vi "Filter and Sort Items.vi"(5 "Sort Info":T5={"Sort Column"=enum."Description", "Ascending?"=FALSE, "Enabled?"=FALSE}, 7 "Filter Info":T7={"Filter Column"=enum."Description", "Filter Type"=enum."Contains", "Filter Value"="", "New Data?"=FALSE, "Enabled?"=FALSE}, 10 "New VI Data":T1[](array[typedef]), 11 "Saved VI Data":T1[](array[typedef])) -> (1 "Displayed Indices":i32[](array[numeric]), 2 "New VI Data out":T1[](array[typedef]), 3 "Saved VI Data out":T1[](array[typedef]))   [LabVIEW 2023, in "VI Properties Editor.lvlib"]
doc: "Filters <B>Saved VI Data</B> according to <B>Filter</B>."
uses:
  VI Properties Editor.lvlib
  CTLs/VI Data.ctl
  CTLs/VI Properties.ctl
  <vilib>/picture/picture.llb/imagedata.ctl
  CTLs/Control Properties.ctl
  CTLs/Filter Info.ctl
  CTLs/Column Name.ctl
  CTLs/Filter Type.ctl
  CTLs/Sort Info.ctl
  <vilib>/regexp/Match Regular Expression.xnode
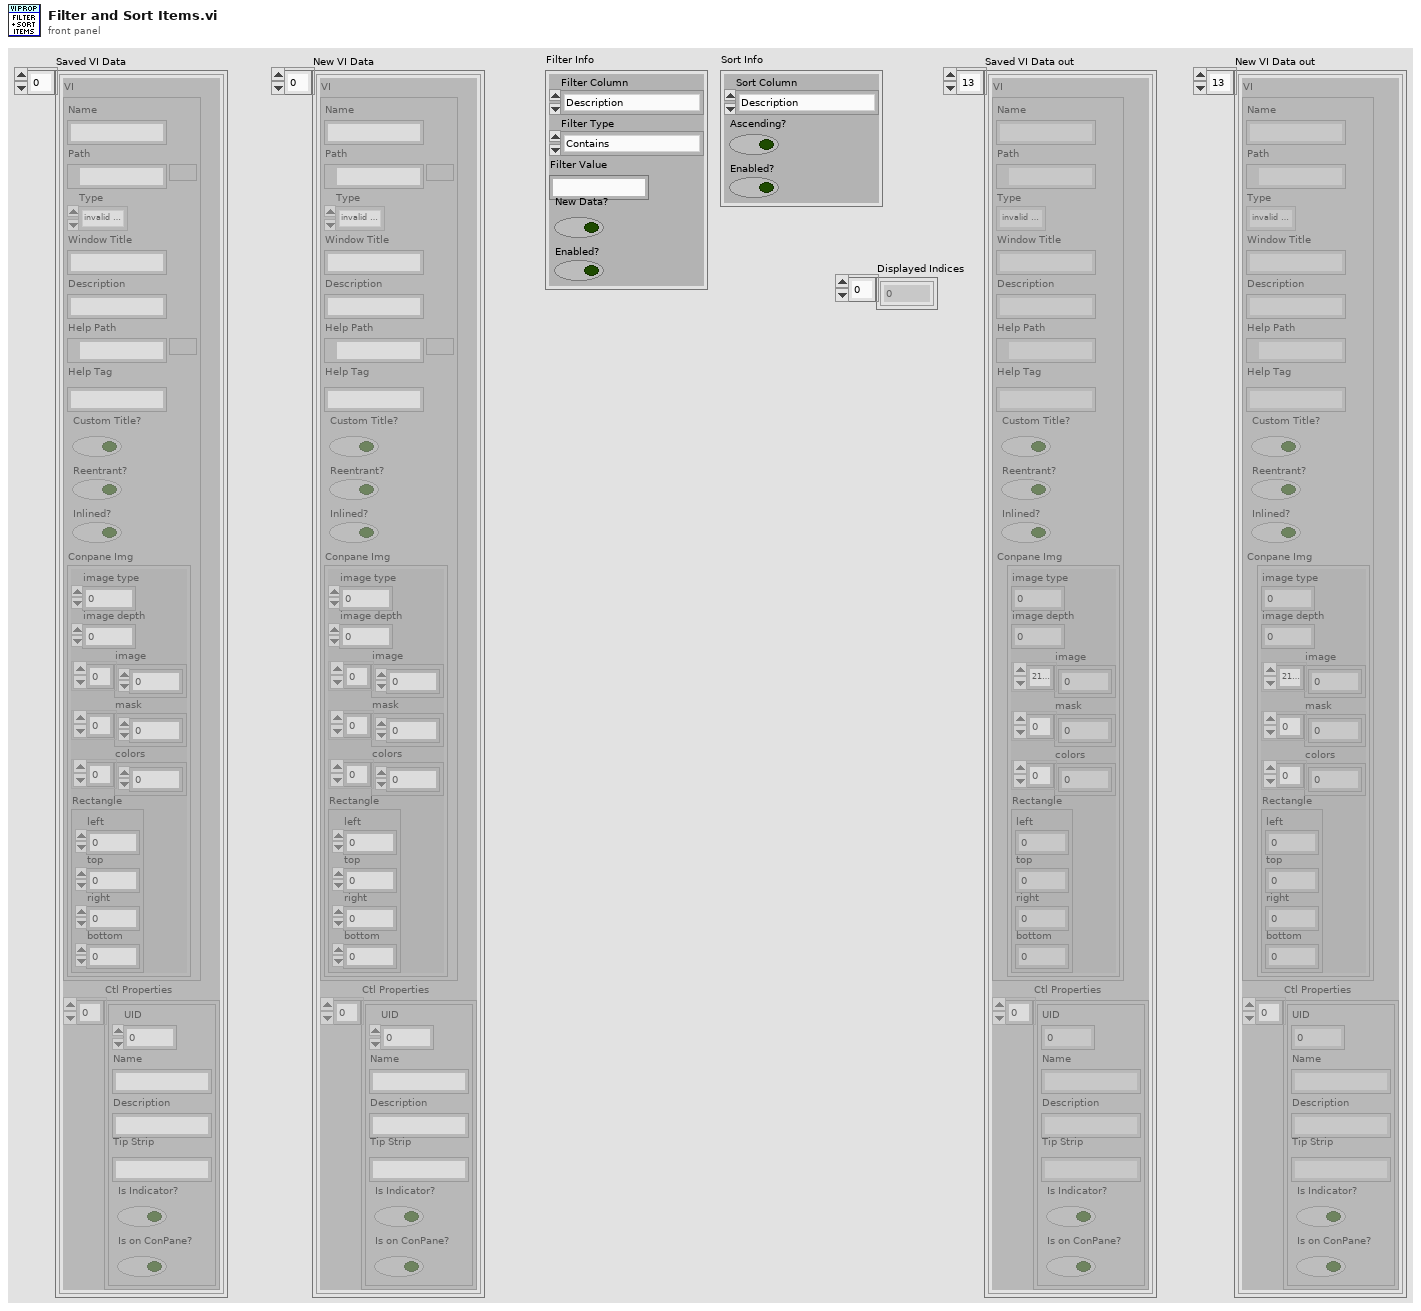
[diagram p1: front panel]
types:
  T1 = typedef "VI Properties Editor.lvlib/VI Data.ctl" = cluster{"VI":T2, "Ctl Properties":T4[]}
  T2 = typedef "VI Properties Editor.lvlib/VI Properties.ctl" = cluster{"Name":string, "Path":path, "Type":enum32{"invalid VI type", "Standard VI", "Control VI", "Global VI", "Polymorphic VI", "Configuration VI", "SubSystem", "Facade VI", "Method VI", "Statechart Diagram VI"}, "Window Title":string, "Description":string, "Help Path":path, "Help Tag":string, "Custom Title?":bool, "Reentrant?":bool, "Inlined?":bool, "Conpane Img":T3}
  T3 = typedef "imagedata.ctl" = cluster{"image type":i32, "image depth":i32, "image":u8[], "mask":u8[], "colors":u32[], "Rectangle":cluster{"left":i16, "top":i16, "right":i16, "bottom":i16}}
  T4 = typedef "VI Properties Editor.lvlib/Control Properties.ctl" = cluster{"UID":i32, "Name":string, "Description":string, "Tip Strip":string, "Is Indicator?":bool, "Is on ConPane?":bool}
  T5 = typedef "VI Properties Editor.lvlib/Sort Info.ctl" = cluster{"Sort Column":T6, "Ascending?":bool, "Enabled?":bool}
  T6 = typedef "VI Properties Editor.lvlib/Column Name.ctl" = enum16{"Name", "Path", "Type", "Window Title", "Description", "Help Path", "Help Tag", "Custom Title?", "Reentrant?", "Inlined?"}
  T7 = typedef "VI Properties Editor.lvlib/Filter Info.ctl" = cluster{"Filter Column":T6, "Filter Type":T8, "Filter Value":string, "New Data?":bool, "Enabled?":bool}
  T8 = typedef "VI Properties Editor.lvlib/Filter Type.ctl" = enum16{"Contains", "Equals", "Starts with", "Ends with", "Does not contain", "Does not equal", "Is empty", "Is not empty"}
  T9 = enum32{"invalid VI type", "Standard VI", "Control VI", "Global VI", "Polymorphic VI", "Configuration VI", "SubSystem", "Facade VI", "Method VI", "Statechart Diagram VI"}
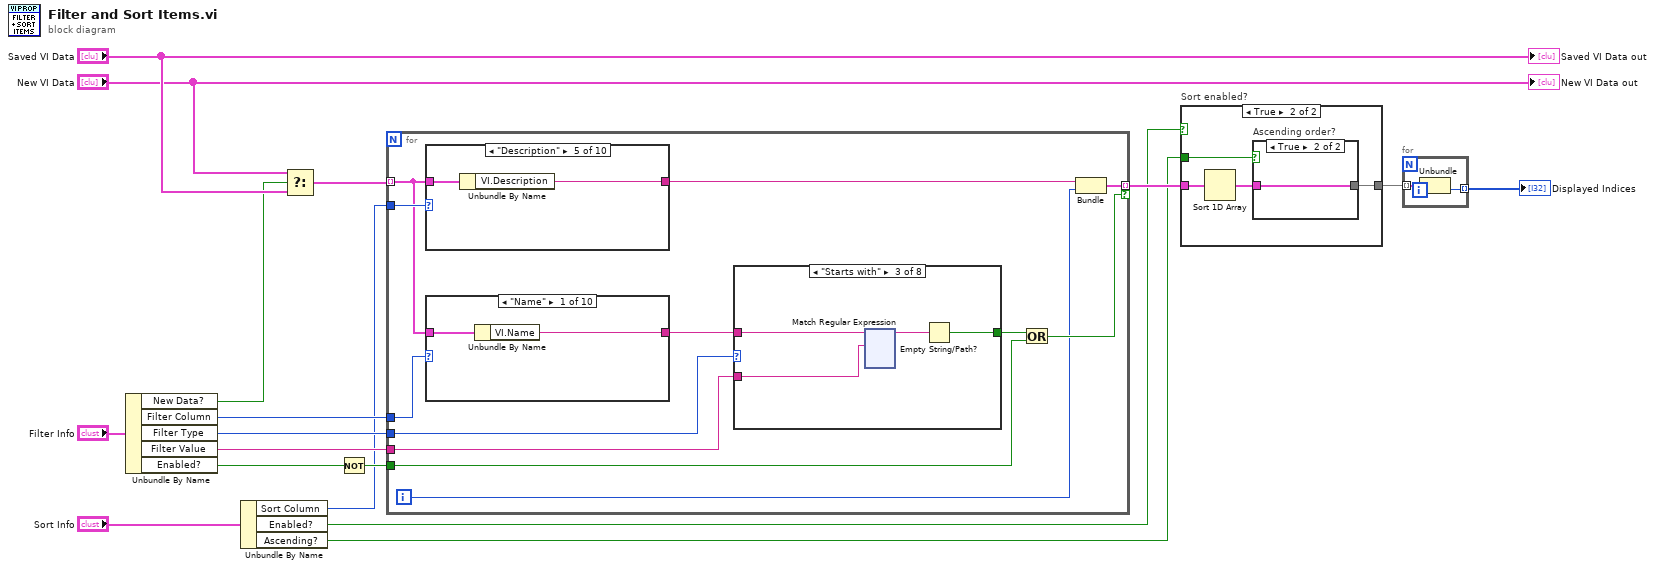
[diagram p0: block diagram]
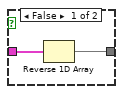
[diagram p3: hidden frame]
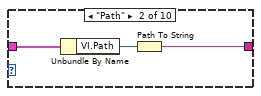
[diagram p4: hidden frame]
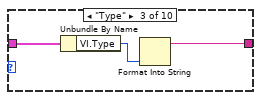
[diagram p5: hidden frame]
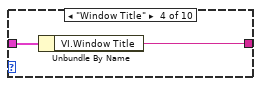
[diagram p6: hidden frame]
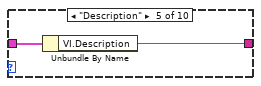
[diagram p7: hidden frame]
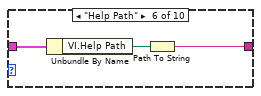
[diagram p8: hidden frame]
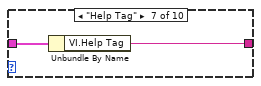
[diagram p9: hidden frame]
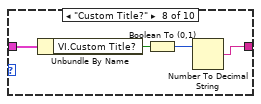
[diagram p10: hidden frame]
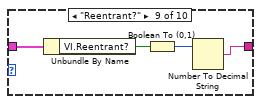
[diagram p11: hidden frame]
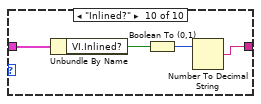
[diagram p12: hidden frame]
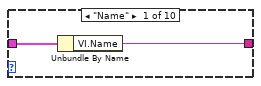
[diagram p13: hidden frame]
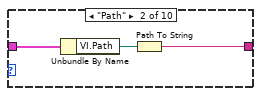
[diagram p14: hidden frame]
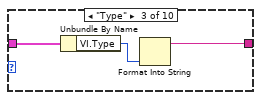
[diagram p15: hidden frame]
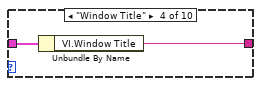
[diagram p16: hidden frame]
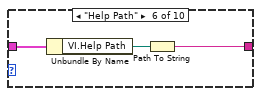
[diagram p17: hidden frame]
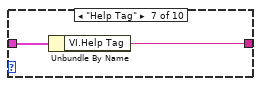
[diagram p18: hidden frame]
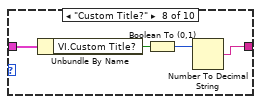
[diagram p19: hidden frame]
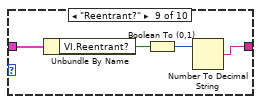
[diagram p20: hidden frame]
diagram:
  n1 = Unbundle By Name("Filter Info") -> ("New Data?"=w3:bool, "Filter Column"=w16:T6, "Filter Type"=w15:T8, "Filter Value"=w14:string, "Enabled?"=w13:bool)
  n2 = Unbundle By Name("Sort Info") -> ("Sort Column"=w7:T6, "Enabled?"=w5:bool, "Ascending?"=w6:bool)
  n3 = Select(t="New VI Data", s=w3, f="Saved VI Data") -> (s? t:f=w2:T1[])
  n4 = Not(x=w13) -> (.not. x?=w12:bool)
  n5 = for {
    tunnel: w2 -> [w20] mode=indexing
    tunnel: w16 -> [w19]
    tunnel: w15 -> [w29]
    tunnel: w14 -> [w28]
    tunnel: [w21] -> w11 mode=indexing if=w26
    tunnel: w12 -> [w25]
    tunnel: w7 -> [w24]
    i -> [w22]
    n6 = case shown="\"Description\"" w24 {
      tunnel: w20 -> [w60 w63 w66 w68 w70 w73 w75 w79 w83 w87]
      tunnel: [w59 w61 w65 w67 w69 w71 w74 w76 w80 w84] -> w23
      frame "Name" {
        n7 = Unbundle By Name(w60) -> ("VI.Name"=w59:string)
      }
      frame "Path" {
        n8 = Unbundle By Name(w63) -> ("VI.Path"=w62:path)
        n9 = Path To String(path=w62) -> (string=w61:string)
      }
      frame "Type" {
        n10 = Unbundle By Name(w66) -> ("VI.Type"=w64:T9)
        n11 = Format Into String(w64) -> (resulting string=w65:string)  [unwired: 3 in, 1 out]
      }
      frame "Window Title" {
        n12 = Unbundle By Name(w68) -> ("VI.Window Title"=w67:string)
      }
      frame "Description" {
        n13 = Unbundle By Name(w70) -> ("VI.Description"=w69:string)
      }
      frame "Help Path" {
        n14 = Unbundle By Name(w73) -> ("VI.Help Path"=w72:path)
        n15 = Path To String(path=w72) -> (string=w71:string)
      }
      frame "Help Tag" {
        n16 = Unbundle By Name(w75) -> ("VI.Help Tag"=w74:string)
      }
      frame "Custom Title?" {
        n17 = Unbundle By Name(w79) -> ("VI.Custom Title?"=w78:bool)
        n18 = Boolean To (0,1)(Boolean=w78) -> (0, 1=w77:i16)
        n19 = Number To Decimal String(number=w77) -> (decimal integer string=w76:string)  [unwired: 1 in]
      }
      frame "Reentrant?" {
        n20 = Unbundle By Name(w83) -> ("VI.Reentrant?"=w82:bool)
        n21 = Boolean To (0,1)(Boolean=w82) -> (0, 1=w81:i16)
        n22 = Number To Decimal String(number=w81) -> (decimal integer string=w80:string)  [unwired: 1 in]
      }
      frame "Inlined?" {
        n23 = Unbundle By Name(w87) -> ("VI.Inlined?"=w86:bool)
        n24 = Boolean To (0,1)(Boolean=w86) -> (0, 1=w85:i16)
        n25 = Number To Decimal String(number=w85) -> (decimal integer string=w84:string)  [unwired: 1 in]
      }
    }
    n26 = case shown="\"Name\"" w19 {
      tunnel: w20 -> [w31 w34 w37 w39 w41 w44 w46 w50 w54 w58]
      tunnel: [w30 w32 w36 w38 w40 w42 w45 w47 w51 w55] -> w18
      frame "Name" {
        n27 = Unbundle By Name(w31) -> ("VI.Name"=w30:string)
      }
      frame "Path" {
        n28 = Unbundle By Name(w34) -> ("VI.Path"=w33:path)
        n29 = Path To String(path=w33) -> (string=w32:string)
      }
      frame "Type" {
        n30 = Unbundle By Name(w37) -> ("VI.Type"=w35:T9)
        n31 = Format Into String(w35) -> (resulting string=w36:string)  [unwired: 3 in, 1 out]
      }
      frame "Window Title" {
        n32 = Unbundle By Name(w39) -> ("VI.Window Title"=w38:string)
      }
      frame "Description" {
        n33 = Unbundle By Name(w41) -> ("VI.Description"=w40:string)
      }
      frame "Help Path" {
        n34 = Unbundle By Name(w44) -> ("VI.Help Path"=w43:path)
        n35 = Path To String(path=w43) -> (string=w42:string)
      }
      frame "Help Tag" {
        n36 = Unbundle By Name(w46) -> ("VI.Help Tag"=w45:string)
      }
      frame "Custom Title?" {
        n37 = Unbundle By Name(w50) -> ("VI.Custom Title?"=w49:bool)
        n38 = Boolean To (0,1)(Boolean=w49) -> (0, 1=w48:i16)
        n39 = Number To Decimal String(number=w48) -> (decimal integer string=w47:string)  [unwired: 1 in]
      }
      frame "Reentrant?" {
        n40 = Unbundle By Name(w54) -> ("VI.Reentrant?"=w53:bool)
        n41 = Boolean To (0,1)(Boolean=w53) -> (0, 1=w52:i16)
        n42 = Number To Decimal String(number=w52) -> (decimal integer string=w51:string)  [unwired: 1 in]
      }
      frame "Inlined?" {
        n43 = Unbundle By Name(w58) -> ("VI.Inlined?"=w57:bool)
        n44 = Boolean To (0,1)(Boolean=w57) -> (0, 1=w56:i16)
        n45 = Number To Decimal String(number=w56) -> (decimal integer string=w55:string)  [unwired: 1 in]
      }
    }
    n46 = case shown="\"Starts with\"" w29 {
      tunnel: w28 -> [w90 w210 w213 w334 _ w458 w578 _]
      tunnel: w18 -> [w91 w211 w215 w336 w455 w459 w579 w581]
      tunnel: [w88 w209 w214 w335 w454 w456 w577 w580] -> w27
      frame "Contains" {
        n47 = xnode "Match Regular Expression"("input string"=w91, "regular expression"=w90) -> ("offset past match"=w89:i32)  [unwired: 4 in, 4 out]
        n48 = Greater Or Equal To 0?(x=w89) -> (x >= 0?=w88:bool)
      }
      frame "Equals" {
        n49 = Equal?(x=w211, y=w210) -> (x = y?=w209:bool)
      }
      frame "Starts with" {
        n50 = xnode "Match Regular Expression"("input string"=w215, "regular expression"=w213) -> ("before match"=w212:string)  [unwired: 4 in, 4 out]
        n51 = Empty String/Path?(string/path=w212) -> (empty?=w214:bool)
      }
      frame "Ends with" {
        n52 = xnode "Match Regular Expression"("input string"=w336, "regular expression"=w334) -> ("after match"=w333:string)  [unwired: 4 in, 4 out]
        n53 = Empty String/Path?(string/path=w333) -> (empty?=w335:bool)
      }
      frame "Is empty" {
        n54 = Empty String/Path?(string/path=w455) -> (empty?=w454:bool)
      }
      frame "Does not contain" {
        n55 = xnode "Match Regular Expression"("input string"=w459, "regular expression"=w458) -> ("offset past match"=w457:i32)  [unwired: 4 in, 4 out]
        n56 = Less Than 0?(x=w457) -> (x < 0?=w456:bool)
      }
      frame "Does not equal" {
        n57 = Not Equal?(x=w579, y=w578) -> (x != y?=w577:bool)
      }
      frame "Is not empty" {
        n58 = Empty String/Path?(string/path=w581) -> (empty?=w580:bool)
      }
    }
    n59 = Or(x=w27, y=w25) -> (x .or. y?=w26:bool)
    n60 = Bundle("Help Tag"=w23, w22) -> (w21:cluster{"Help Tag":string, i32})  [unwired: 1 in]
  }
  n61 = case "Sort enabled?" shown="True" w5 {
    tunnel: w11 -> [w582 w586]
    tunnel: [w582 w584] -> w10
    tunnel: w6 -> [_ w583]
    frame False {
    }
    frame True {
      n62 = Sort 1D Array(array=w586) -> (sorted array=w585:cluster{"Help Tag":string, i32}[])
      n63 = case "Ascending order?" shown="True" w583 {
        tunnel: w585 -> [w588 w589]
        tunnel: [w587 w589] -> w584
        frame False {
          n64 = Reverse 1D Array(array=w588) -> (reversed array=w587:cluster{"Help Tag":string, i32}[])
        }
        frame True {
        }
      }
    }
  }
  n65 = for {
    tunnel: w10 -> [w591] mode=indexing
    tunnel: [w590] -> w9 mode=indexing
    n66 = Unbundle(w591) -> (w590:i32)  [unwired: 1 out]
  }
  "Displayed Indices" <- w9
  "Saved VI Data out" <- "Saved VI Data"
  "New VI Data out" <- "New VI Data"
